vi "sensor cmd calibration data blob.vi"(9 "dest_length":i32, 10 "dest":string, 11 "device_handle":u32) -> (1 "function return":i32, 2 "dest out":string, 3 "device_handle out":u32)   [LabVIEW 2019, in "apdm.lvlib"]
doc: "APDM_EXPORT int apdm_sensor_cmd_calibration_data_blob(apdm_device_handle_t device_handle, uint8_t *dest, const int dest_length);"
uses:
  apdm.lvlib
  Lee Lab/CP FES Walking 2018/Code/Working/LabVIEW/apdm.dll
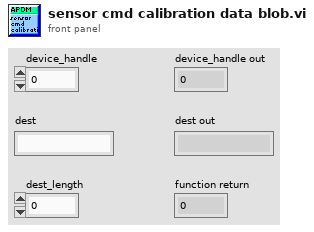
[diagram p1: front panel]
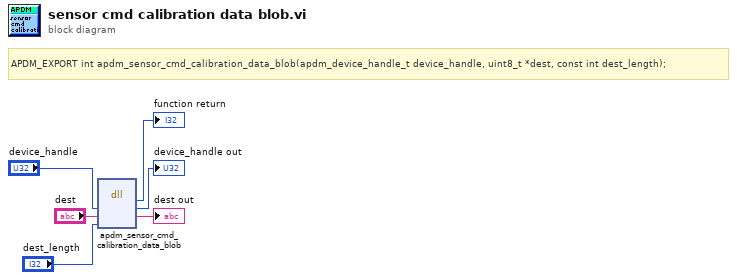
[diagram p0: block diagram]
diagram:
  # "APDM_EXPORT int apdm_sensor_cmd_calibration_data_blob(apdm_device_handle_t device_handle, uint8_t *dest, const int dest_length);"
  n1 = dll-call lib="C:/Users/jfalesi/Dropbox/Lee Lab/CP FES Walking 2018/Code/Working/LabVIEW/apdm.*" fn="apdm_sensor_cmd_calibration_data_blob"("device_handle"="device_handle", "dest"="dest", "dest_length"="dest_length") -> (→"function return":i32, "device_handle"=→"device_handle out":u32, "dest"=→"dest out":string)  [unwired: 4 in, 2 out]
